vi "DSF.Engine.Framework.Get Hardware Info.vi"(11 "Framework in":refnum<class "DSF.Engine.Framework.lvclass">) -> (2 "Hardware Info":refnum<class "DSF.Engine.Hardware Info.lvclass">, 3 "Framework out":refnum<class "DSF.Engine.Framework.lvclass">)   [LabVIEW 2017, in "DSF.Engine.lvlib" / "DSF.Engine.Framework.lvclass"]
uses:
  DSF.Engine.Framework.lvclass
  Hardware/DSF.Engine.Hardware Info.lvclass
  DSF.Engine.Framework.lvclass/DSF.Engine.Framework.ctl
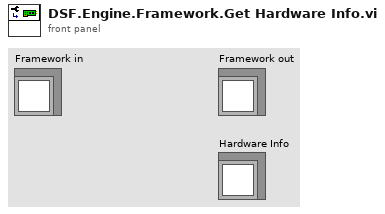
[diagram p1: front panel]
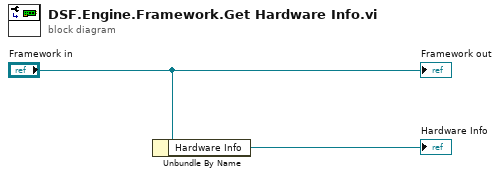
[diagram p0: block diagram]
diagram:
  n1 = Unbundle By Name("Framework in") -> ("Hardware Info"=→"Hardware Info":refnum<class "DSF.Engine.Hardware Info.lvclass">)
  "Framework out" <- "Framework in"
